vi "Data to BMS Status.vi"(1 "Data":u8[](array[numeric])) -> (0 "BMS Status":T1)   [LabVIEW 2016]
uses:
  Tests/BMS Status.ctl
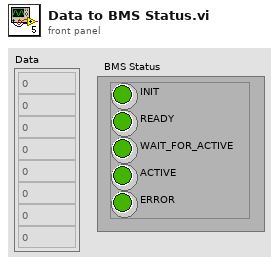
[diagram p1: front panel]
types:
  T1 = typedef "BMS Status.ctl" = cluster{"INIT":bool, "READY":bool, "WAIT_FOR_ACTIVE":bool, "ACTIVE":bool, "ERROR":bool}
  T2 = cluster{"Boolean array[0]":bool, "Boolean array[1]":bool, "Boolean array[2]":bool, "Boolean array[3]":bool, "Boolean array[4]":bool}
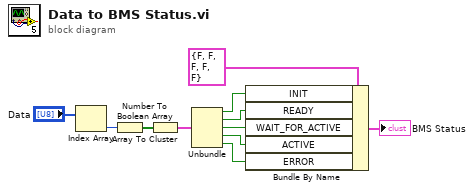
[diagram p0: block diagram]
diagram:
  n1 = Index Array(array="Data") -> (element=w8:u8)  [unwired: 1 in]
  n2 = Number To Boolean Array(number=w8) -> (Boolean array=w7:bool[])
  n3 = Array To Cluster(array=w7) -> (cluster=w6:T2)
  n4 = Unbundle(w6) -> ("Boolean array[0]"=w5:bool, "Boolean array[1]"=w4:bool, "Boolean array[2]"=w3:bool, "Boolean array[3]"=w2:bool, "Boolean array[4]"=w1:bool)
  n5 = Bundle By Name(cluster=T1 {"INIT"=FALSE, "READY"=FALSE, "WAIT_FOR_ACTIVE"=FALSE, "ACTIVE"=FALSE, "ERROR"=FALSE} ("BMS Status"), "INIT"=w5, "READY"=w4, "WAIT_FOR_ACTIVE"=w3, "ACTIVE"=w2, "ERROR"=w1) -> (→"BMS Status":T1)
